vi "UDP_Inquiry-Bin.vi"(10 "IN_Param":string) -> (2 "Inquiry":T1 {"Sens"."ID2" format="%.0x"; "Sens"."ID1" format="%.0x"; "AmpUnit" format="%.0x"; "AnalogCH" format="%.0x"; "USB" format="%.0x"; "IP_Busy" format="%.0x"; "Count" format="%.0x"; "IP"."D" format="%.0x"; "IP"."C" format="%.0x"; "IP"."B" format="%.0x"; "IP"."A" format="%.0x"})   [LabVIEW 2017]
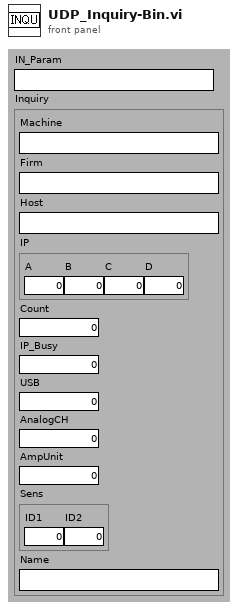
[diagram p1: front panel]
types:
  T1 = cluster{"Machine":string, "Firm":string, "Host":string, "IP":cluster{"A":u8, "B":u8, "C":u8, "D":u8}, "Count":u32, "IP_Busy":u32, "USB":u32, "AnalogCH":u32, "AmpUnit":u32, "Sens":cluster{"ID1":u16, "ID2":u16}, "Name":string}
  T2 = cluster{"IN_Param":string, "IN_Param":string, "IN_Param":string, cluster{u8, u8, u8, u8}, "dimension size":u32, "dimension size":u32, "dimension size":u32, "dimension size":u32, "dimension size":u32, "output cluster":cluster{u16, u16}, "IN_Param":string}
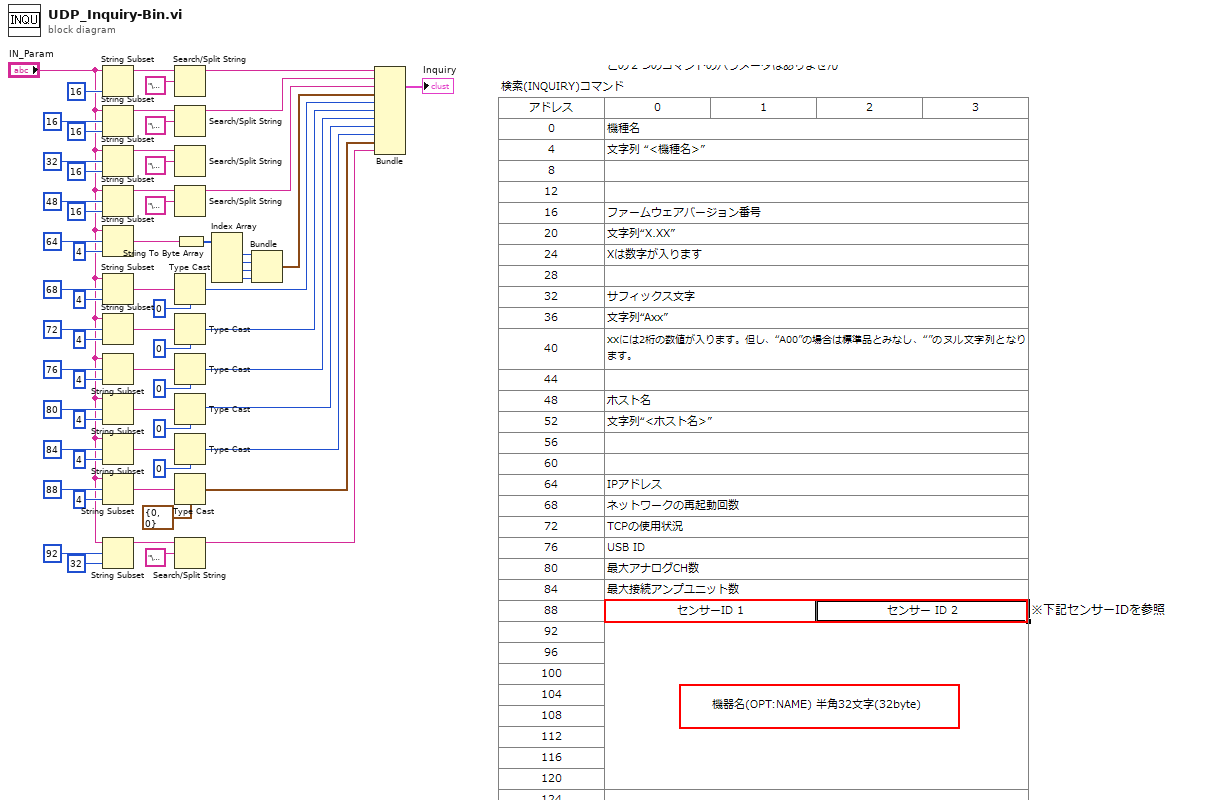
[diagram p0: block diagram]
diagram:
  (unwired) u32 0 ("dimension size")
  n1 = String Subset(string="IN_Param", length (rest)=16 ("length (rest)")) -> (substring=w52:string)  [unwired: 1 out]
  n2 = String Subset(string="IN_Param", offset (0)=16, length (rest)=16 ("length (rest)")) -> (substring=w46:string)
  n3 = String Subset(string="IN_Param", offset (0)=32, length (rest)=16 ("length (rest)")) -> (substring=w47:string)
  n4 = String Subset(string="IN_Param", offset (0)=48, length (rest)=16 ("length (rest)")) -> (substring=w48:string)
  n5 = String Subset(string="IN_Param", offset (0)=64, length (rest)=4 ("length (rest)")) -> (substring=w39:string)
  n6 = String Subset(string="IN_Param", offset (0)=68, length (rest)=4 ("length (rest)")) -> (substring=w44:string)
  n7 = String Subset(string="IN_Param", offset (0)=72, length (rest)=4 ("length (rest)")) -> (substring=w32:string)
  n8 = String Subset(string="IN_Param", offset (0)=76, length (rest)=4 ("length (rest)")) -> (substring=w25:string)
  n9 = String Subset(string="IN_Param", offset (0)=80, length (rest)=4 ("length (rest)")) -> (substring=w24:string)
  n10 = String Subset(string="IN_Param", offset (0)=84, length (rest)=4 ("length (rest)")) -> (substring=w17:string)
  n11 = String Subset(string="IN_Param", offset (0)=88, length (rest)=4 ("length (rest)")) -> (substring=w16:string)
  n12 = String Subset(string="IN_Param", offset (0)=92, length (rest)=32 ("length (rest)")) -> (substring=w8:string)
  n13 = Search/Split String(string=w52, search string/char (-)="\u0000") -> (substring before match=w43:string)  [unwired: 3 out]
  n14 = Search/Split String(string=w46, search string/char (-)="\u0000") -> (substring before match=w42:string)  [unwired: 3 out]
  n15 = Search/Split String(string=w47, search string/char (-)="\u0000") -> ()  [unwired: 4 out]
  n16 = Search/Split String(string=w48, search string/char (-)="\u0000") -> (substring before match=w41:string)  [unwired: 3 out]
  n17 = Type Cast(type=u32 0 ("dimension size"), x=w44) -> (*(type *) &x=w7:u32)
  n18 = Type Cast(type=u32 0 ("dimension size"), x=w32) -> (*(type *) &x=w6:u32)
  n19 = Type Cast(type=u32 0 ("dimension size"), x=w25) -> (*(type *) &x=w5:u32)
  n20 = Type Cast(type=u32 0 ("dimension size"), x=w24) -> (*(type *) &x=w4:u32)
  n21 = Type Cast(type=u32 0 ("dimension size"), x=w17) -> (*(type *) &x=w3:u32)
  n22 = Type Cast(type=cluster{u16, u16} {0, 0} ("output cluster"), x=w16) -> (*(type *) &x=w2:cluster{u16, u16})
  n23 = Search/Split String(string=w8, search string/char (-)="\u0000") -> (substring before match=w1:string)  [unwired: 3 out]
  n24 = String To Byte Array(string=w39) -> (unsigned byte array=w38:u8[])
  n25 = Index Array(array=w38) -> (element #1=w37:u8, element #2=w36:u8, element #3=w35:u8, element #4=w34:u8)  [unwired: 4 in]
  n26 = Bundle(w37, w36, w35, w34) -> (w33:cluster{u8, u8, u8, u8})  [unwired: 1 out]
  n27 = Bundle("IN_Param"=w43, "IN_Param"=w42, "IN_Param"=w41, w33, "dimension size"=w7, "dimension size"=w6, "dimension size"=w5, "dimension size"=w4, "dimension size"=w3, "output cluster"=w2, "IN_Param"=w1) -> (→"Inquiry":T2)  [unwired: 1 out]
